vi "File Indexer.vi"(11 "File Index In":i32) -> (3 "File Indicator Out":string)   [LabVIEW 2018]
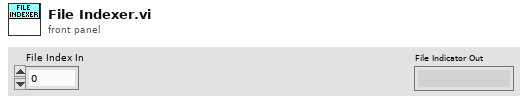
[diagram p1: front panel]
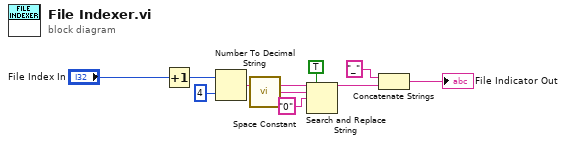
[diagram p0: block diagram]
diagram:
  n1 = Increment(x="File Index In") -> (x+1=w10:i32)
  n2 = Number To Decimal String(number=w10, width (-)=i16 4) -> (decimal integer string=w8:string)
  n3 = call <vilib>:"Space Constant.vi"() -> ("String"=w7:string)
  n4 = Search and Replace String(replace all?=TRUE ("replace all? (F)"), input string=w8, search string=w7, replace string="0" ("replace string (\"\")")) -> (result string=w3:string)  [unwired: 4 in, 3 out]
  n5 = Concatenate Strings("_", w3) -> (→"File Indicator Out":string)
